vi "Write Config.vi"(8 "error in (no error)":errorcluster, 10 "Config":T1, 11 "Path":path) -> (0 "error out":errorcluster)   [LabVIEW 2023, in "VI Properties Editor.lvlib"]
doc: "Writes to a config file located at <B>Path</B>."
uses:
  VI Properties Editor.lvlib
  <vilib>/Utility/config.llb/NI_LVConfig.lvlib
  <vilib>/Utility/config.llb/Write Key (Boolean).vi
  <vilib>/Utility/config.llb/Write Key (String).vi
  CTLs/Config.ctl
  CTLs/Column Name.ctl
  CTLs/Filter Type.ctl
  CTLs/Filter Info.ctl
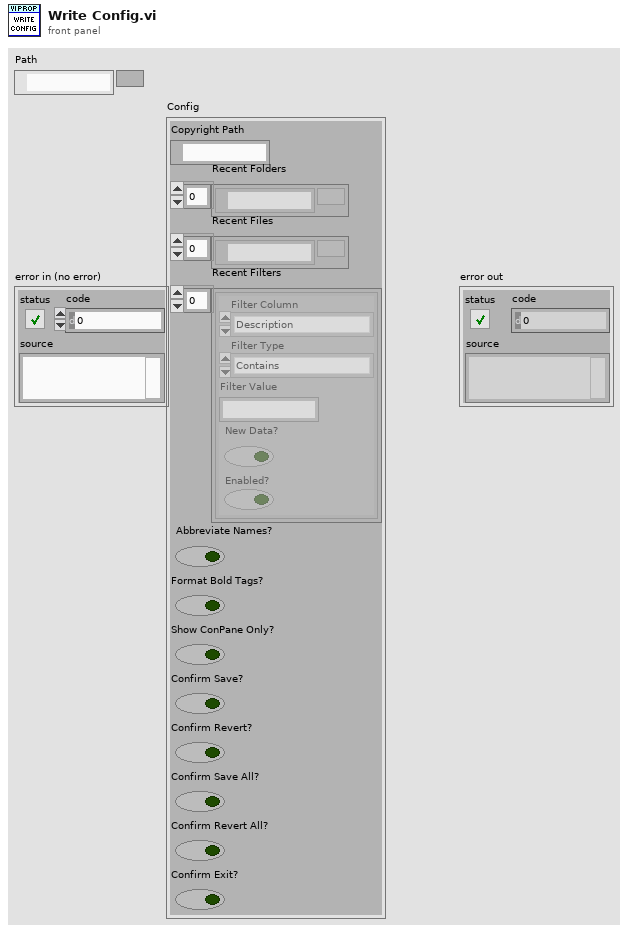
[diagram p1: front panel]
types:
  T1 = typedef "VI Properties Editor.lvlib/Config.ctl" = cluster{"Copyright Path":path, "Recent Folders":path[], "Recent Files":path[], "Recent Filters":T2[], "Abbreviate Names?":bool, "Format Bold Tags?":bool, "Show ConPane Only?":bool, "Confirm Save?":bool, "Confirm Revert?":bool, "Confirm Save All?":bool, "Confirm Revert All?":bool, "Confirm Exit?":bool}
  T2 = typedef "VI Properties Editor.lvlib/Filter Info.ctl" = cluster{"Filter Column":T3, "Filter Type":T4, "Filter Value":string, "New Data?":bool, "Enabled?":bool}
  T3 = typedef "VI Properties Editor.lvlib/Column Name.ctl" = enum16{"Name", "Path", "Type", "Window Title", "Description", "Help Path", "Help Tag", "Custom Title?", "Reentrant?", "Inlined?"}
  T4 = typedef "VI Properties Editor.lvlib/Filter Type.ctl" = enum16{"Contains", "Equals", "Starts with", "Ends with", "Does not contain", "Does not equal", "Is empty", "Is not empty"}
  T5 = typedef "NI_LVConfig.lvlib/Config Data RefNum.ctl" = refnum<k1>
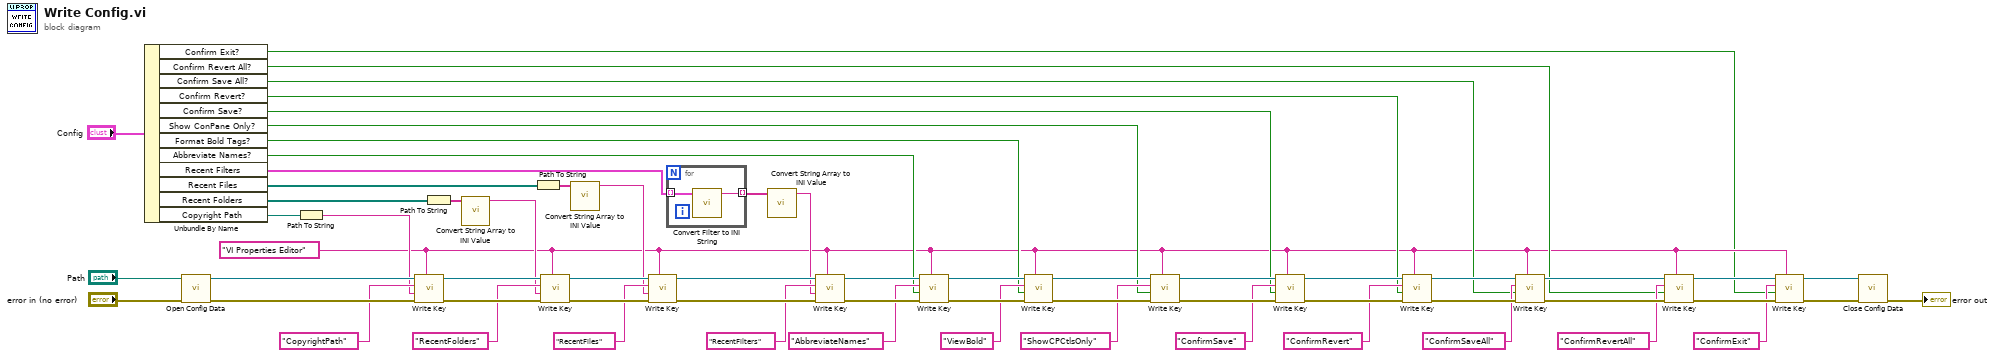
[diagram p0: block diagram]
diagram:
  w2 = "VI Properties Editor" ("section")
  n1 = Unbundle By Name("Config") -> ("Confirm Exit?"=w1:bool, "Confirm Revert All?"=w13:bool, "Confirm Save All?"=w14:bool, "Confirm Revert?"=w15:bool, "Confirm Save?"=w16:bool, "Show ConPane Only?"=w25:bool, "Format Bold Tags?"=w39:bool, "Abbreviate Names?"=w40:bool, "Recent Filters"=w10:T2[], "Recent Files"=w29:path[], "Recent Folders"=w32:path[], "Copyright Path"=w41:path)
  n2 = call <vilib>:"Open Config Data.vi"("error in (no error)"="error in (no error)", "configuration file path"="Path") -> ("error out"=w58:errorcluster, "refnum"=w46:T5)  [unwired: 7 in, 1 out]
  n3 = Path To String(path=w41) -> (string=w37:string)
  n4 = call-poly <vilib>:"Write Key.vi"("section"=w2, "error in (no error)"=w58, "value"=w37, "key"="CopyrightPath", "refnum"=w46) -> ("error out"=w54:errorcluster, "refnum out"=w33:T5)  [unwired: 4 in, 1 out]
  n5 = Path To String(path=w32) -> (string=w31:string[])
  n6 = call "Convert String Array to INI Value.vi"("String Array"=w31) -> ("INI Value"=w12:string)  [unwired: 10 in]
  n7 = Path To String(path=w29) -> (string=w30:string[])
  n8 = call-poly <vilib>:"Write Key.vi"("section"=w2, "error in (no error)"=w54, "value"=w12, "key"="RecentFolders", "refnum"=w33) -> ("error out"=w53:errorcluster, "refnum out"=w34:T5)  [unwired: 4 in, 1 out]
  n9 = call "Convert String Array to INI Value.vi"("String Array"=w30) -> ("INI Value"=w28:string)  [unwired: 10 in]
  n10 = call-poly <vilib>:"Write Key.vi"("section"=w2, "error in (no error)"=w53, "value"=w28, "key"="RecentFiles", "refnum"=w34) -> ("error out"=w52:errorcluster, "refnum out"=w11:T5)  [unwired: 4 in, 1 out]
  n11 = for {
    tunnel: w10 -> [w64] mode=indexing
    tunnel: [w63] -> w9 mode=indexing
    n12 = call "Convert Filter to INI String.vi"("Filter Info"=w64) -> ("INI String"=w63:string)  [unwired: 10 in]
  }
  n13 = call "Convert String Array to INI Value.vi"("String Array"=w9) -> ("INI Value"=w7:string)  [unwired: 10 in]
  n14 = call-poly <vilib>:"Write Key.vi"("section"=w2, "error in (no error)"=w52, "value"=w7, "key"="RecentFilters", "refnum"=w11) -> ("error out"=w61:errorcluster, "refnum out"=w60:T5)  [unwired: 4 in, 1 out]
  n15 = call-poly <vilib>:"Write Key.vi"("section"=w2, "error in (no error)"=w61, "value"=w40, "key"="AbbreviateNames", "refnum"=w60) -> ("error out"=w55:errorcluster, "refnum out"=w43:T5)  [unwired: 4 in, 1 out]
  n16 = call-poly <vilib>:"Write Key.vi"("section"=w2, "error in (no error)"=w55, "value"=w39, "key"="ViewBold", "refnum"=w43) -> ("error out"=w57:errorcluster, "refnum out"=w27:T5)  [unwired: 4 in, 1 out]
  n17 = call-poly <vilib>:"Write Key.vi"("section"=w2, "error in (no error)"=w57, "value"=w25, "key"="ShowCPCtlsOnly", "refnum"=w27) -> ("error out"=w49:errorcluster, "refnum out"=w20:T5)  [unwired: 4 in, 1 out]
  n18 = call-poly <vilib>:"Write Key.vi"("section"=w2, "error in (no error)"=w49, "value"=w16, "key"="ConfirmSave", "refnum"=w20) -> ("error out"=w51:errorcluster, "refnum out"=w19:T5)  [unwired: 4 in, 1 out]
  n19 = call-poly <vilib>:"Write Key.vi"("section"=w2, "error in (no error)"=w51, "value"=w15, "key"="ConfirmRevert", "refnum"=w19) -> ("error out"=w48:errorcluster, "refnum out"=w18:T5)  [unwired: 4 in, 1 out]
  n20 = call-poly <vilib>:"Write Key.vi"("section"=w2, "error in (no error)"=w48, "value"=w14, "key"="ConfirmSaveAll", "refnum"=w18) -> ("error out"=w50:errorcluster, "refnum out"=w17:T5)  [unwired: 4 in, 1 out]
  n21 = call-poly <vilib>:"Write Key.vi"("section"=w2, "error in (no error)"=w50, "value"=w13, "key"="ConfirmRevertAll", "refnum"=w17) -> ("error out"=w62:errorcluster, "refnum out"=w4:T5)  [unwired: 4 in, 1 out]
  n22 = call-poly <vilib>:"Write Key.vi"("section"=w2, "error in (no error)"=w62, "value"=w1, "key"="ConfirmExit", "refnum"=w4) -> ("error out"=w5:errorcluster, "refnum out"=w3:T5)  [unwired: 4 in, 1 out]
  n23 = call <vilib>:"Close Config Data.vi"("error in (no error)"=w5, "refnum"=w3) -> ("error out"=→"error out":errorcluster)  [unwired: 8 in, 1 out]
